vi "Process.vi"(11 "Base jettl in":refnum<class "Base jettl.lvclass">) -> (3 "Base jettl out":refnum<class "Base jettl.lvclass">)   [LabVIEW 2021, in "jettl.lvlib" / "Base jettl.lvclass"]
uses:
  Base jettl.lvclass
  Base jettl.lvclass/Base jettl.ctl
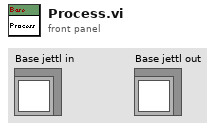
[diagram p1: front panel]
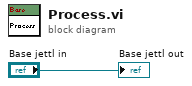
[diagram p0: block diagram]
diagram:
  "Base jettl out" <- "Base jettl in"
